vi "Read Called From Msg Library.vi"(11 "Base Teller in":refnum<class "Base Teller.lvclass">) -> (2 "Called From Msg Library":bool)   [LabVIEW 2020, in "jettl.lvlib" / "Base Teller.lvlib" / "Base Teller.lvclass"]
uses:
  Base Teller.lvclass
  Base Teller.lvclass/Base Teller.ctl
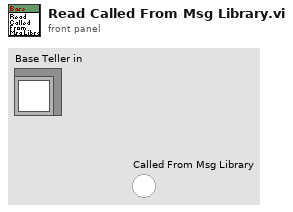
[diagram p1: front panel]
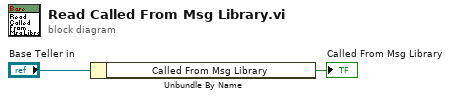
[diagram p0: block diagram]
diagram:
  n1 = Unbundle By Name("Base Teller in") -> ("Called From Msg Library"=→"Called From Msg Library":bool)
